vi "Calculate Particle Scores Ball.vi"(10 "Sorted Data":dbl[][](array[numeric])) -> (3 "Scores":T1[](array[typedef]))   [LabVIEW 2019]
doc: "Calculate scores based on the particle measurements. Calculated scores are for aspect ratio, area to convex hull area, and moment of inertia. These scores range between 0 and 100 and can be used to categorize particles as targets and non-targets."
uses:
  Target Fields.ctl
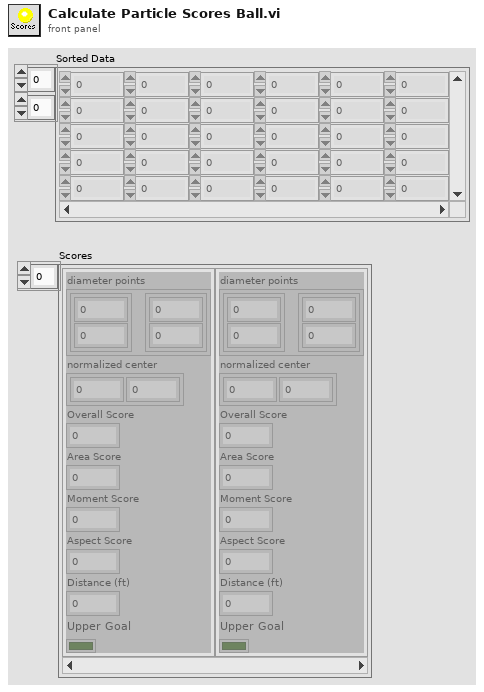
[diagram p1: front panel]
types:
  T1 = typedef "Target Fields.ctl" = cluster{"diameter points":cluster{"first point":cluster{"x":dbl, "y":dbl}, "projected point":cluster{"x":dbl, "y":dbl}}, "normalized center":cluster{"x":dbl, "y":dbl}, "Overall Score":dbl, "Area Score":dbl, "Moment Score":dbl, "Aspect Score":dbl, "Distance (ft)":dbl, "Upper Goal":bool}
  T2 = cluster{cluster{"Numeric":dbl, "Numeric":dbl}, cluster{"Numeric":dbl, "Numeric":dbl}}
  T3 = cluster{cluster{cluster{"Numeric":dbl, "Numeric":dbl}, cluster{"Numeric":dbl, "Numeric":dbl}}, "first point":cluster{"x":dbl, "y":dbl}, dbl, "Score":dbl, "Score":dbl, "Score":dbl, dbl, bool}
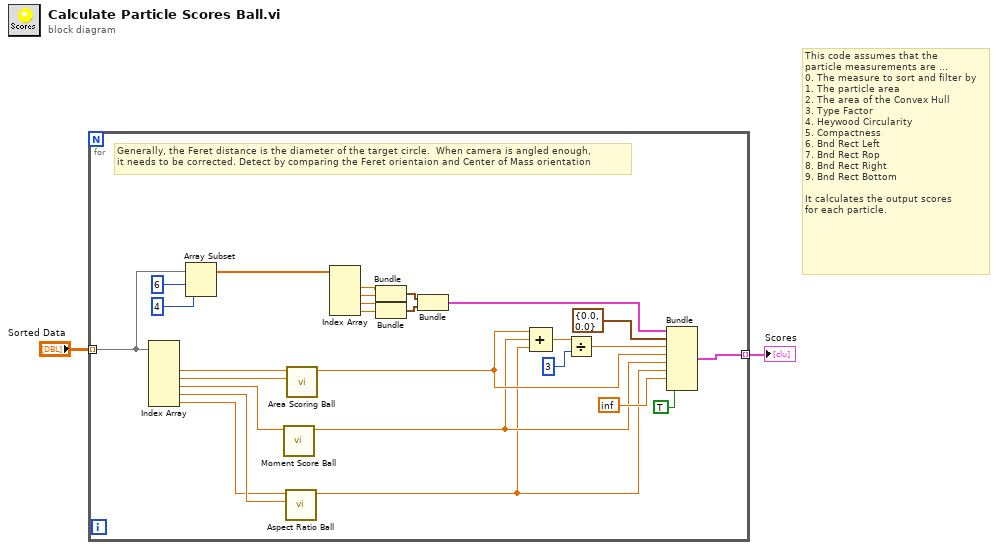
[diagram p0: block diagram]
diagram:
  # "This code assumes that the\nparticle measurements are ...\n0. The measure to sort and filter by\n1. The particle area\n2. The area of the Convex Hull\n3. Type Factor\n4. Heywood Circularity\n5. Compactness\n6. Bnd Rect Left\n7. Bnd Rect Rop\n8. Bnd Rect Right\n9. Bnd Rect Bottom\n\nIt calculates the output scores\nfor each particle."
  n1 = for {
    tunnel: "Sorted Data" -> [w19] mode=indexing
    tunnel: [w17] -> w1 mode=indexing
    # "Generally, the Feret distance is the diameter of the target circle.  When camera is angled enough,\nit needs to be corrected. Detect by comparing the Feret orientaion and Center of Mass orientation"
    n2 = Index Array(array=w19) -> (element #2=w10:dbl, element #3=w5:dbl, element #4=w7:dbl, element #5=w4:dbl, element #6=w3:dbl)  [unwired: 6 in, 1 out]
    n3 = Array Subset(array=w19, index=6, length=4) -> (w26:dbl[])
    n4 = call "Moment Score Ball.vi"("Moment Factor"=w7) -> ("Score"=w8:dbl)  [unwired: 10 in]
    n5 = call "Aspect Ratio Ball.vi"("Circularity"=w4, "Compactness"=w3) -> ("Score"=w6:dbl)  [unwired: 9 in]
    n6 = call "Area Scoring Ball.vi"("Convex Hull Area"=w5, "Area"=w10) -> ("Score"=w9:dbl)  [unwired: 9 in]
    n7 = Index Array(array=w26) -> (element #1=w13:dbl, element #2=w14:dbl, element #3=w15:dbl, element #4=w16:dbl)  [unwired: 4 in]
    n8 = Bundle("Numeric"=w13, "Numeric"=w14) -> (w12:cluster{"Numeric":dbl, "Numeric":dbl})  [unwired: 1 in]
    n9 = Bundle("Numeric"=w15, "Numeric"=w16) -> (w11:cluster{"Numeric":dbl, "Numeric":dbl})  [unwired: 1 in]
    n10 = Bundle(w12, w11) -> (w22:T2)  [unwired: 1 in]
    n11 = Compound Arithmetic op=ADD(w9, w8, w6) -> (w24:dbl)
    n12 = Divide(x=w24, y=3) -> (x/y=w18:dbl)
    n13 = Bundle(w22, "first point"=cluster{"x":dbl, "y":dbl} {"x"=0.0, "y"=0.0}, w18, "Score"=w9, "Score"=w8, "Score"=w6, inf, TRUE) -> (w17:T3)  [unwired: 1 in]
  }
  "Scores" <- w1
